vi "Ryans Arrange.vi"(6 "Variant in":variant, 7 "Shift Pressed?":bool, 8 "error in (no error)":errorcluster, 10 "QD Combo Box Ref":refnum<vi>, 11 "QD Launch VI Ref":refnum<vi>) -> (0 "error out":errorcluster, 4 "Variant out":variant)   [LabVIEW 2019]
doc: "Arranges the block diagram or front panel objects depending on the selection:\n\nFP + No Selection:\n Arranges all controls and indicators by relative position, snaps to grid and resets the panel origins.\n\nFP + Selection:\n Arranges the selected controls by the left edge and snaps to grid. \n Hold Shift to arrange the selected controls by the top edge.\n\nBD + No Selection:\n Arranges all terminals to the adjacent terminal and align controls/indicators left/right respectively.\n\nBD + Selection:\n Arranges the selected objects to adjacent terminal (left-to-right). \n Hold Shift to arrange the selection in reverse order (right-to-left).\n Note: Constants are arranged relative to the adjacent terminal position.\n\nCreated by: Ryan Pacini\n\nDefault Shortcut - [A]"
uses:
  _Script/Scripts/_Builtins/Builtins.lvlib
  _Script/Script.lvlib
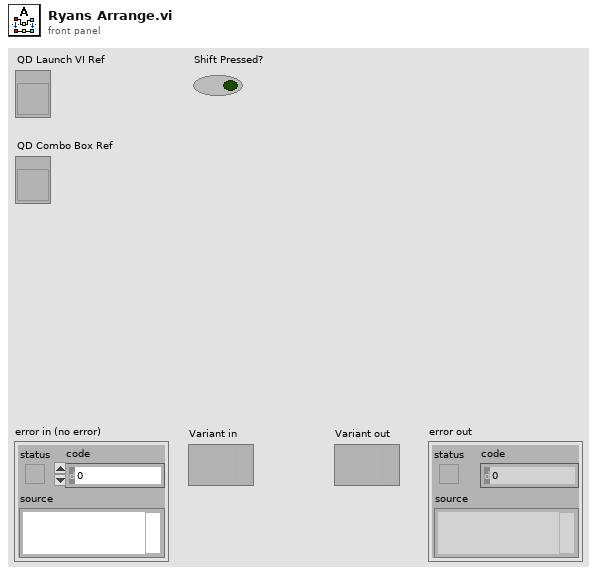
[diagram p1: front panel]
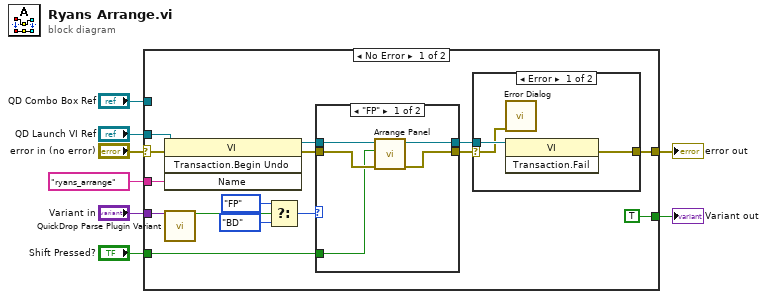
[diagram p0: block diagram]
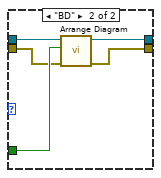
[diagram p2: hidden frame]
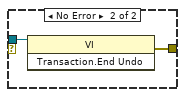
[diagram p3: hidden frame]
diagram:
  n1 = case shown="No Error" "error in (no error)" {
    selector: "error in (no error)" -> [w23 w39]
    tunnel: [w22 w39] -> w3
    tunnel: "QD Launch VI Ref" -> [w18 _]
    tunnel: "ryans_arrange" ("Undo Name") -> [w21 _]
    tunnel: "Variant in" -> [w19 _]
    tunnel: [TRUE _] -> w4
    tunnel: "QD Combo Box Ref" -> [_ _]
    tunnel: "Shift Pressed?" -> [w9 _]
    frame No Error {
      n2 = invoke class="VI" method="Transaction.Begin Undo"(reference=w18, error in=w23, "Name"=w21) -> (reference out=w17:refnum<vi>, error out=w16:errorcluster)  [unwired: 1 in, 2 out]
      n3 = call <vilib>:"QuickDrop Parse Plugin Variant.vi"("QDKS Variant in"=w19) -> ("QD Launch VI Panel?"=w11:bool)  [unwired: 12 in, 2 out]
      n4 = Select(t=enum8{"FP", "BD"}."FP" ("Panel"), s=w11, f=enum8{"FP", "BD"}."BD" ("Panel")) -> (s? t:f=w10:enum8{"FP", "BD"})
      n5 = case shown="\"FP\"" w10 {
        tunnel: w17 -> [w25 w30]
        tunnel: w16 -> [w27 w29]
        tunnel: [w28 w33] -> w15
        tunnel: [w26 w32] -> w14
        tunnel: w9 -> [w24 w31]
        frame "FP" {
          n6 = call "Arrange Panel.vi"("error in (no error)"=w27, "Shift?"=w24, "VI Refnum in"=w25) -> ("error out"=w28:errorcluster, "VI Refnum out"=w26:refnum<vi>)  [unwired: 7 in]
        }
        frame "BD" {
          n7 = call "Arrange Diagram.vi"("error in (no error)"=w29, "Shift?"=w31, "VI Refnum in"=w30) -> ("error out"=w33:errorcluster, "VI Refnum out"=w32:refnum<vi>)  [unwired: 7 in]
        }
      }
      n8 = case shown="Error" w15 {
        selector: w15 -> [w34 _]
        tunnel: w14 -> [w35 w37]
        tunnel: [w36 w38] -> w22
        frame Error {
          n9 = call "Error Dialog.vi"("error in (no error)"=w34) -> ()  [unwired: 9 in, 2 out]
          n10 = invoke class="VI" method="Transaction.Fail"(reference=w35) -> (error out=w36:errorcluster)  [unwired: 2 in, 2 out]
        }
        frame No Error {
          n11 = invoke class="VI" method="Transaction.End Undo"(reference=w37) -> (error out=w38:errorcluster)  [unwired: 2 in, 2 out]
        }
      }
    }
    frame Error {
    }
  }
  "error out" <- w3
  "Variant out" <- w4
